vi "RP IV analysis.vi"() -> ()   [LabVIEW 2016]
uses:
  RP Core/Rep Pitaya I-V driver/RP I-V Configuration.ctl
  Waform generation/I-V parameters.ctl
panel:
  in  "RP I-V Configuration":T1={"I-V parameters"={"Start magnitude"=0.0, "Magnitude increment"=0.0, "End magnitude"=0.0, "Baseline length"=0, "Ramp length"=0, "Top  length"=0, "Threshold "=0.0, "Processing delay"=0, "Valhalla range"=0.0, "Interpolation"=0}, "Ranges"=[], "Pre-trigger duration"=0.01, "Post-trigger duration"=0.1, "Output delay"=0.1} {"Output delay" format="%#_6ps"; "Post-trigger duration" format="%#_6ps"; "Pre-trigger duration" format="%#_6ps"; "Ranges" format="%#_6pV"; "I-V parameters"."Valhalla range" format="%#_6pA"; "I-V parameters"."Processing delay" format="%dpts"; "I-V parameters"."Threshold" format="%#_6pV"; "I-V parameters"."Top  length" format="%dpts"; "I-V parameters"."Ramp length" format="%dpts"; "I-V parameters"."Baseline length" format="%dpts"; "I-V parameters"."End magnitude" format="%#_6pA"; "I-V parameters"."Magnitude increment" format="%#_6pA"; "I-V parameters"."Start magnitude" format="%#_6pA"}
  in  "Save?":bool
  in  "Clip":i32=17
  out "Iv curves 2":cluster{dbl[], dbl[]}(graph)
  in  "Current resistor":dbl=1.0 format="%#_13g"
  in  "Slicing threshold":dbl format="%#_6p"
  in  "Preamp\nsetting I":dbl=10.0 format="x%#_6p"
  in  "Preamp\nsetting V":dbl=500.0 format="x%#_6p"
  in  "Invert V":bool
  in  "Invert I":bool
  out "Iv curves":T3(graph)
  out "Current vs Time":dbl[](graph)
  in  "Current Channel":string="I"
  out "Voltage vs Time":dbl[](graph)
  in  "Voltage Channel":string="V"
  in  "Delay":dbl=-0.000445 format="%#_6p"
  in  "File Path":path
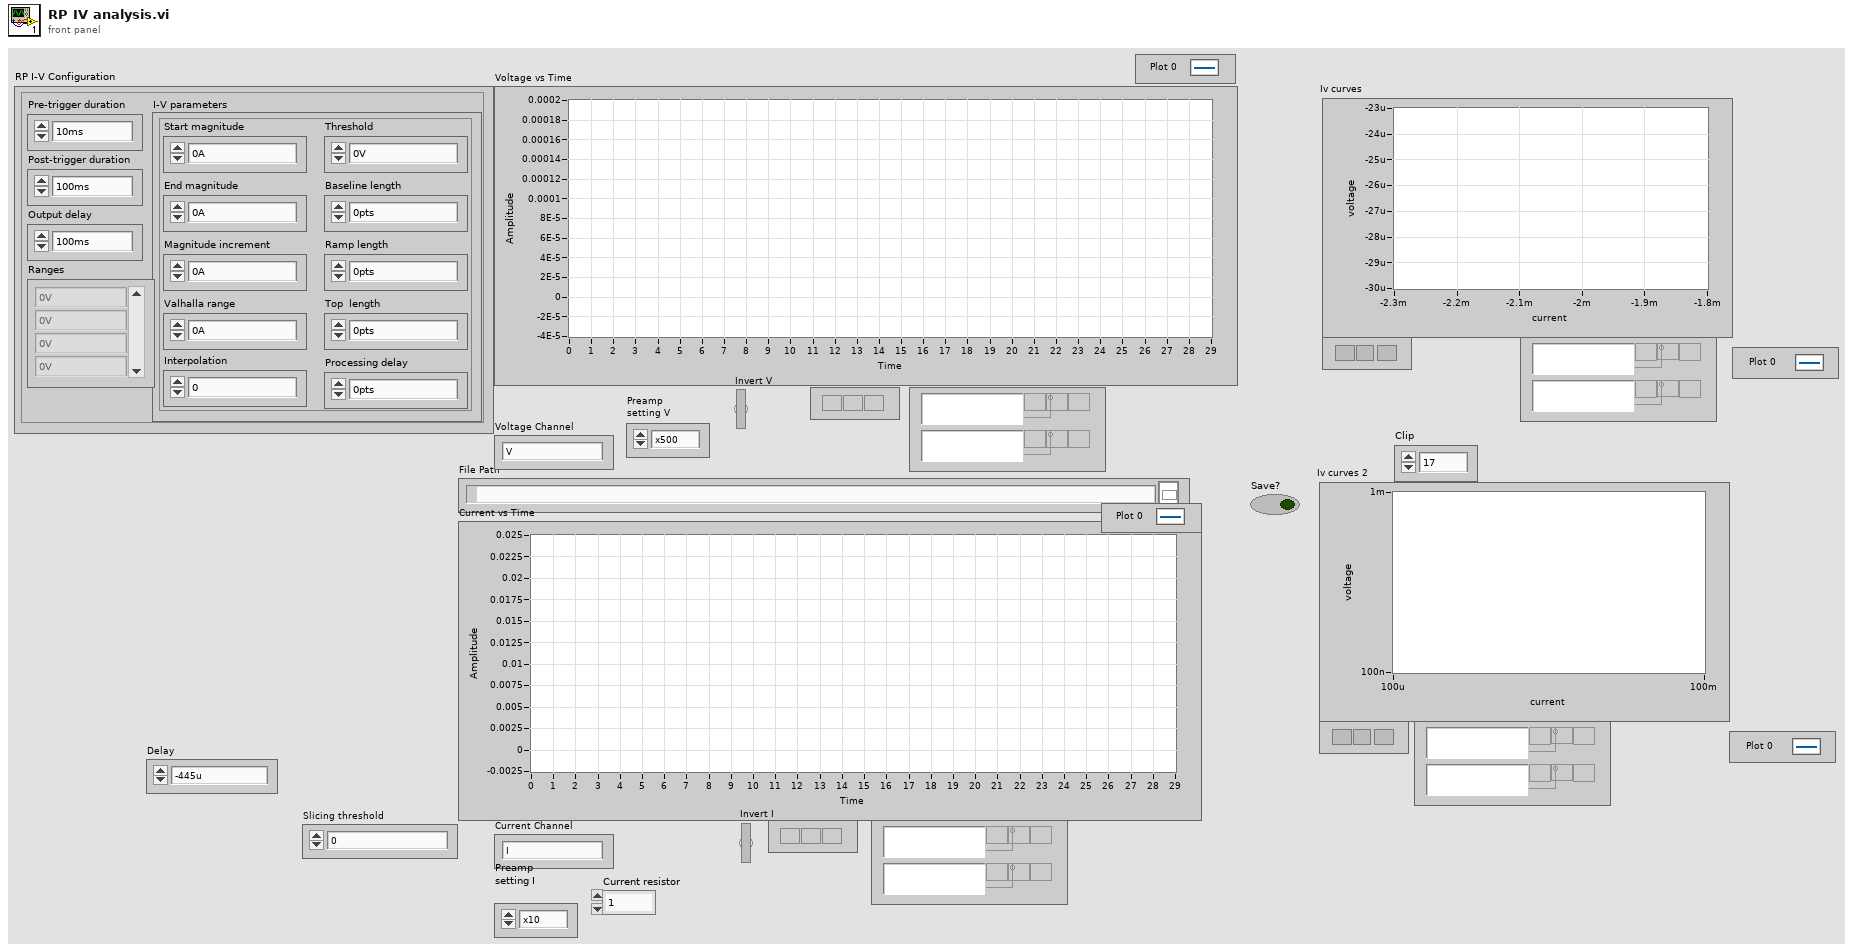
[diagram p1: front panel]
types:
  T1 = typedef "RP I-V Configuration.ctl" = cluster{"I-V parameters":T2, "Ranges":dbl[], "Pre-trigger duration":dbl, "Post-trigger duration":dbl, "Output delay":dbl}
  T2 = typedef "I-V parameters.ctl" = cluster{"Start magnitude":dbl, "Magnitude increment":dbl, "End magnitude":dbl, "Baseline length":i32, "Ramp length":i32, "Top  length":i32, "Threshold ":dbl, "Processing delay":u16, "Valhalla range":dbl, "Interpolation":i32}
  T3 = cluster{"Sliced array":dbl[], "Sliced array":dbl[]}[]
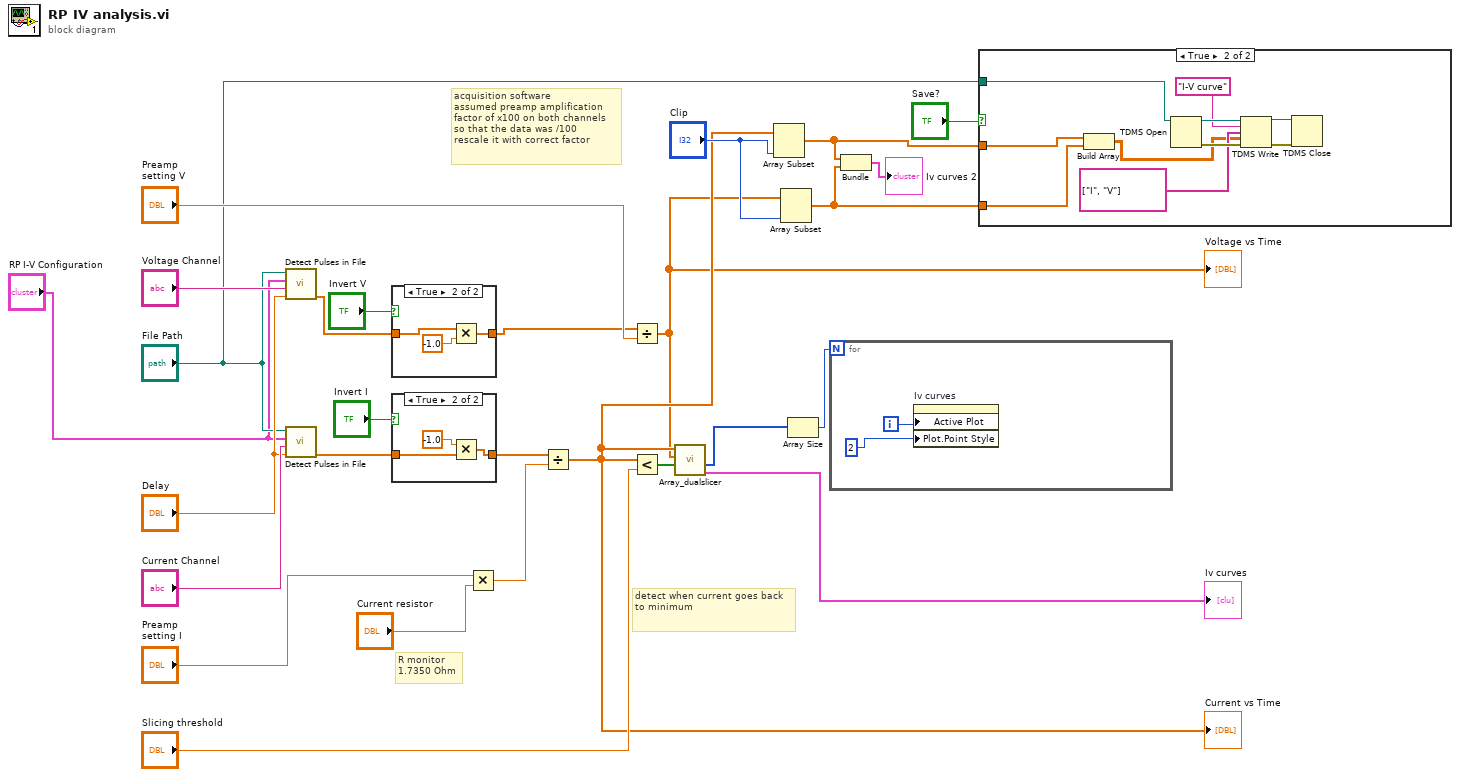
[diagram p0: block diagram]
diagram:
  # "detect when current goes back to minimum"
  # "R monitor\n1.7350 Ohm"
  # "acquisition software\nassumed preamp amplification\nfactor of x100 on both channels\nso that the data was /100\nrescale it with correct factor"
  n1 = call "Detect Pulses in File.vi"("Delay"="Delay", "Channel name"="Voltage Channel", "RP I-V Configuration"="RP I-V Configuration", "File Path"="File Path") -> ("Avg signal minus\nAvg background"=w22:dbl[])  [unwired: 5 in, 2 out]
  n2 = call "Detect Pulses in File.vi"("Delay"="Delay", "Channel name"="Current Channel", "RP I-V Configuration"="RP I-V Configuration", "File Path"="File Path") -> ("Avg signal minus\nAvg background"=w19:dbl[])  [unwired: 5 in, 2 out]
  n3 = case shown="True" "Invert V" {
    tunnel: w22 -> [w28 w31]
    tunnel: [w28 w29] -> w20
    frame False {
    }
    frame True {
      n4 = Multiply(x=w31, y=-1.0) -> (x*y=w29:dbl[])
    }
  }
  n5 = case shown="True" "Invert I" {
    tunnel: [w32 w34] -> w16
    tunnel: w19 -> [w32 w33]
    frame False {
    }
    frame True {
      n6 = Multiply(x=-1.0, y=w33) -> (x*y=w34:dbl[])
    }
  }
  n7 = Multiply(x="Preamp\nsetting I", y="Current resistor") -> (x*y=w17:dbl)
  n8 = Divide(x=w16, y=w17) -> (x/y=w8:dbl[])
  "Current vs Time" <- w8
  n9 = Divide(x=w20, y="Preamp\nsetting V") -> (x/y=w7:dbl[])
  "Voltage vs Time" <- w7
  n10 = Less?(x=w8, y="Slicing threshold") -> (x < y?=w13:bool[])
  n11 = call "Array_dualslicer.vi"("X array"=w8, "Y array"=w7, "Slicing array"=w13) -> ("Lengths"=w11:i32[], "Output cluster"=→"Iv curves":cluster{dbl[], dbl[]}[])  [unwired: 1 in, 4 out]
  n12 = Array Subset(array=w8, length="Clip") -> (w3:dbl[])  [unwired: 1 in]
  n13 = Array Subset(array=w7, length="Clip") -> (w2:dbl[])  [unwired: 1 in]
  n14 = Array Size(array=w11) -> (size(s)=w10:i32)
  n15 = for {
    N: w10 -> [_]
    i -> [w37]
    n16 = property on="Iv curves" class="XYGraph (strict)"("Active Plot"=w37, "Plot.Point Style"=u8 2) -> ()  [unwired: 2 in, 2 out]
  }
  n17 = Bundle(w3, w2) -> (→"Iv curves 2":cluster{dbl[], dbl[]})  [unwired: 1 in]
  n18 = case shown="True" "Save?" {
    tunnel: "File Path" -> [_ w47]
    tunnel: w3 -> [_ w40]
    tunnel: w2 -> [_ w39]
    frame False {
    }
    frame True {
      n19 = Build Array(w40, w39) -> (w38:dbl[][])
      n20 = TDMS Open(11:w47) -> (0:w45:errorcluster, 3:w46:refnum<k34>)  [unwired: 6 in]
      n21 = TDMS Write(0:w46, 5:"I-V curve" ("group name in (Untitled)"), 7:string[] ["I", "V"] ("channel name(s) in (Untitled)"), 9:w38, 11:w45) -> (4:w43:refnum<k34>, 15:w44:errorcluster)  [unwired: 1 in, 2 out]
      n22 = TDMS Close(8:w44, 11:w43) -> ()  [unwired: 2 out]
    }
  }
